vi "Get Window Position (left, top).vi"(0 "VI in":refnum<vi>) -> (4 "VI out":refnum<vi>, 8 "left, top":cluster{"Left":i16, "Top":i16}, 15 "error out":errorcluster)   [LabVIEW 2020]
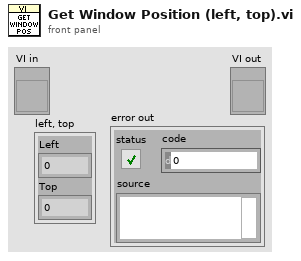
[diagram p1: front panel]
types:
  T1 = typedef "LVRectTypeDef.ctl" = cluster{"Left":i16, "Top":i16, "Right":i16, "Bottom":i16}
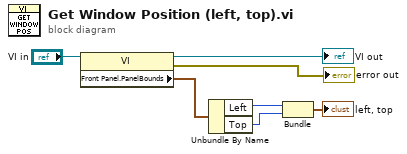
[diagram p0: block diagram]
diagram:
  n1 = property class="VI"(reference="VI in") -> (reference out=→"VI out":refnum<vi>, error out=→"error out":errorcluster, "Front Panel.PanelBounds"=w7:T1)  [unwired: 1 in]
  n2 = Unbundle By Name(w7) -> ("Left"=w3:i16, "Top"=w2:i16)
  n3 = Bundle("Left"=w3, "Top"=w2) -> (→"left, top":cluster{"Left":i16, "Top":i16})  [unwired: 1 in]
